vi "ingresaMediciones.vi"(8 "error in (no error)":errorcluster, 9 "fila tabla":i32, 10 "max value":dbl, 11 "Prueba08 in":refnum<class "Prueba08.lvclass">) -> (0 "error out":errorcluster, 3 "Prueba08 out":refnum<class "Prueba08.lvclass">)   [LabVIEW 2019, in "Prueba08.lvclass"]
uses:
  Prueba08.lvclass
  Prueba08.lvclass/Prueba08.ctl
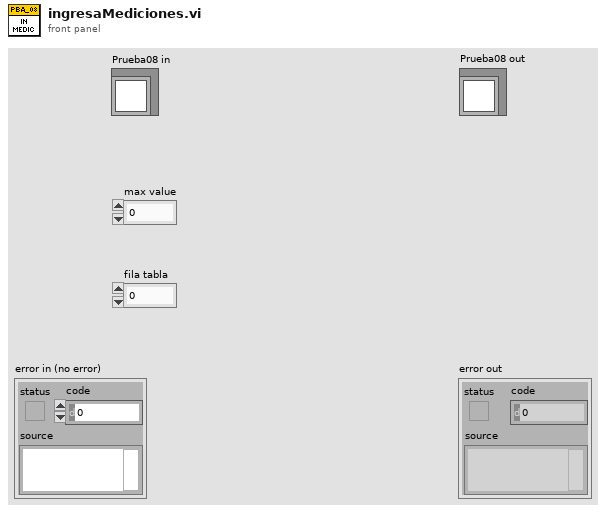
[diagram p1: front panel]
types:
  T1 = cluster{"Medido":dbl, "Error":dbl, "Ref":dbl, "Incert_exp":dbl, "Tol+":dbl, "Tol-":dbl, "fila":i32}
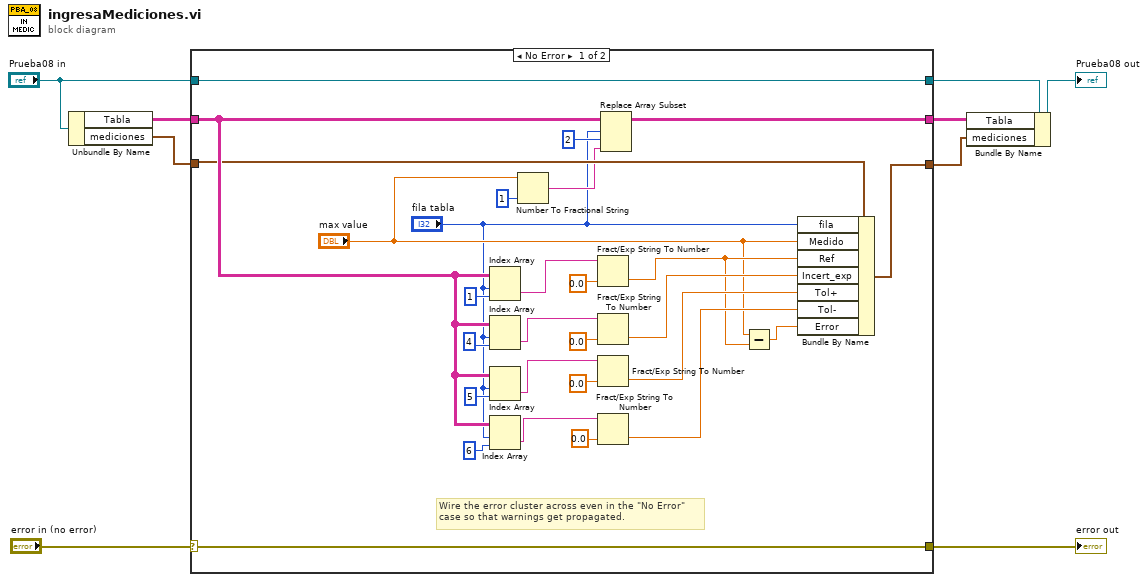
[diagram p0: block diagram]
diagram:
  n1 = Unbundle By Name("Prueba08 in") -> ("Tabla"=w5:string[][], "mediciones"=w4:T1)
  n2 = case shown="No Error" "error in (no error)" {
    selector: "error in (no error)" -> [w36 w41]
    tunnel: [w36 w41] -> w8
    tunnel: [w37 w40] -> w7
    tunnel: "Prueba08 in" -> [w37 w40]
    tunnel: w5 -> [w19 w39]
    tunnel: w4 -> [w18 w38]
    tunnel: [w17 w39] -> w2
    tunnel: [w16 w38] -> w1
    frame No Error {
      # "Wire the error cluster across even in the \"No Error\"\ncase so that warnings get propagated."
      n3 = Index Array(array=w19, index (row)="fila tabla", index (col)=1 ("disabled index (col)")) -> (element=w33:string)
      n4 = Index Array(array=w19, index (row)="fila tabla", index (col)=4 ("index (row)")) -> (element=w29:string)
      n5 = Index Array(array=w19, index (row)="fila tabla", index (col)=5 ("disabled index (col)")) -> (element=w20:string)
      n6 = Index Array(array=w19, index (row)="fila tabla", index (col)=6 ("index (row)")) -> (element=w23:string)
      n7 = Number To Fractional String(number="max value", precision (6)=i16 1) -> (F-format string=w11:string)  [unwired: 2 in]
      n8 = Fract/Exp String To Number(string=w33, default (0 dbl)=0.0) -> (number=w15:dbl)  [unwired: 2 in, 1 out]
      n9 = Fract/Exp String To Number(string=w29, default (0 dbl)=0.0) -> (number=w28:dbl)  [unwired: 2 in, 1 out]
      n10 = Fract/Exp String To Number(string=w20, default (0 dbl)=0.0) -> (number=w21:dbl)  [unwired: 2 in, 1 out]
      n11 = Fract/Exp String To Number(string=w23, default (0 dbl)=0.0) -> (number=w22:dbl)  [unwired: 2 in, 1 out]
      n12 = Replace Array Subset(array=w19, new element=w11, index (row)="fila tabla", index (col)=2 ("disabled index (col)")) -> (w17:string[][])
      n13 = Subtract(x="max value", y=w15) -> (x-y=w14:dbl)
      n14 = Bundle By Name(cluster=w18, "fila"="fila tabla", "Medido"="max value", "Ref"=w15, "Incert_exp"=w28, "Tol+"=w21, "Tol-"=w22, "Error"=w14) -> (w16:T1)
    }
    frame Error {
    }
  }
  "error out" <- w8
  n15 = Bundle By Name(cluster=w7, "Tabla"=w2, "mediciones"=w1) -> (→"Prueba08 out":refnum<class "Prueba08.lvclass">)
